vi "Receive.vi"(8 "error in (no error)":errorcluster, 10 "Transfer Group in":refnum<class "Transfer Group.lvclass">, 11 "DSFPlugin in":refnum<class "DSFPlugin Transceiver.lvclass">) -> (0 "error out":errorcluster, 2 "Transfer Group out":refnum<class "Transfer Group.lvclass">, 3 "DSFPlugin out":refnum<class "DSFPlugin Transceiver.lvclass">)   [LabVIEW 2017, in "DSFPluginTest.lvlib" / "DSFPlugin Transceiver.lvclass"]
uses:
  DSFPlugin Transceiver.lvclass
  builds/Data Sharing Framework/Current/Data Sharing Framework Core/DSF Core.lvlibp/Engine/Classes/Transfer Group/Transfer Group.lvclass
  DSFPlugin Transceiver.lvclass/DSFPlugin Transceiver.ctl
  builds/Data Sharing Framework/Current/Data Sharing Framework Core/DSF Core.lvlibp/Engine/Classes/Transceiver/Transceiver.lvclass
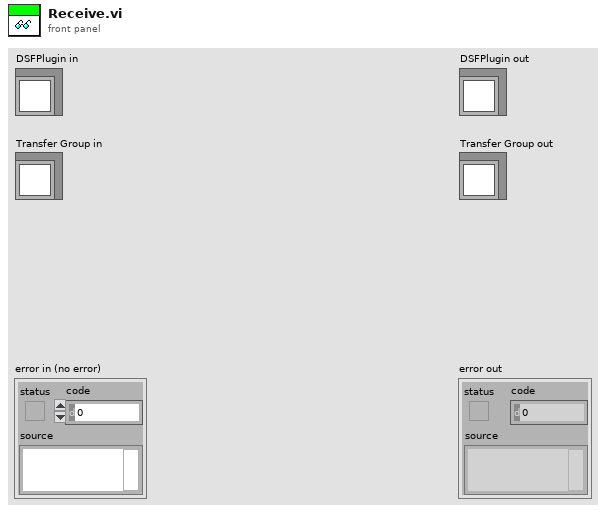
[diagram p1: front panel]
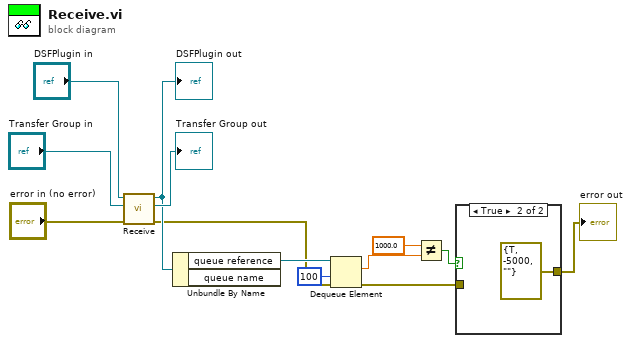
[diagram p0: block diagram]
diagram:
  n1 = call-parent "Receive.vi"("error in (no error)"="error in (no error)", "Transfer Group in"="Transfer Group in", "Transceiver in"="DSFPlugin in") -> ("error out"=w7:errorcluster, "Transfer Group out"=→"Transfer Group out":refnum<class "Transfer Group.lvclass">, "Transceiver out"=w9:refnum<class "DSFPlugin Transceiver.lvclass">)  [unwired: 6 in]
  "DSFPlugin out" <- w9
  n2 = Unbundle By Name(w9) -> ("queue reference"=w8:refnum<queue>)  [unwired: 1 out]
  n3 = Dequeue Element(queue=w8, timeout in ms (-1)=100, error in (no error)=w7) -> (element=w6:dbl, error out=w2:errorcluster)  [unwired: 2 out]
  n4 = Not Equal?(x=1000.0, y=w6) -> (x != y?=w4:bool)
  n5 = case shown="True" w4 {
    tunnel: [w14 errorcluster {"status"=TRUE, "code"=-5000, "source"=""} ("error constant")] -> w3
    tunnel: w2 -> [w14 _]
    frame False {
    }
    frame True {
    }
  }
  "error out" <- w3
